vi "Test Dog Bark.vi"(8 "error in (no error)":errorcluster, 11 "Dog Test In":refnum<class "Dog Test.lvclass">) -> (0 "error out":errorcluster, 3 "Dog Test Out":refnum<class "Dog Test.lvclass">)   [LabVIEW 2020, in "Dog Test.lvclass"]
doc: "Test Dog bark"
uses:
  Dog Test.lvclass
  C:/Program Files (x86)/National Instruments/LabVIEW 2020/vi.lib/Astemes/LUnit/Test Case.lvclass
  <vilib>/Astemes/LUnit/Test Case.lvclass/Test Case.ctl
  600ed3a1-22d3-4fb8-9d64-ca09b61efaae.vi
  <vilib>/Astemes/LUnit/Append Pass Result.vi
  <vilib>/Astemes/LUnit/Append Fail Result.vi
  <vilib>/Astemes/LUnit/Describe Comparison.vi
  <vilib>/Astemes/LUnit/Compare Variants.vi
  <vilib>/Astemes/LUnit/Run In UI.vi
  <vilib>/Utility/error.llb/Clear Errors.vi
  <vilib>/Astemes/LUnit/Describe Variant.vi
  Animal Classes/Dog/Dog.lvclass
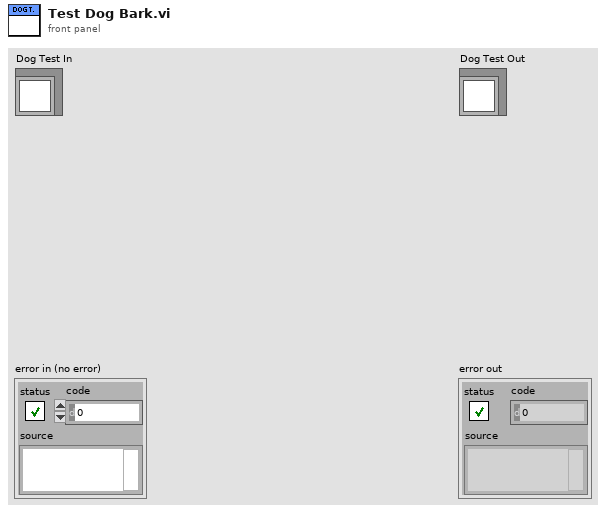
[diagram p1: front panel]
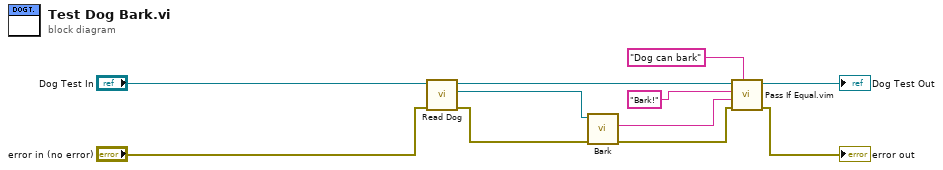
[diagram p0: block diagram]
diagram:
  n1 = call "Read Dog.vi"("error in (no error)"="error in (no error)", "Dog Test in"="Dog Test In") -> ("error out"=w8:errorcluster, "Dog.lvclass"=w9:refnum<class "Dog.lvclass">, "Dog Test out"=w7:refnum<class "Dog Test.lvclass">)  [unwired: 7 in]
  n2 = call "Bark.vi"("error in (no error)"=w8, "Dog In"=w9) -> ("error out"=w2:errorcluster, "Result"=w4:string)  [unwired: 7 in, 1 out]
  n3 = call "Pass If Equal.vim"("Description"="Dog can bark", "error in (no error)"=w2, "Actual"=w4, "Expected"="Bark!", "LUnit Test Case In"=w7) -> ("error out"=→"error out":errorcluster, "LUnit Test Case Out"=→"Dog Test Out":refnum<class "Dog Test.lvclass">)  [unwired: 5 in]
